vi "forceSubpanelAbort.vi"(8 "error in":errorcluster, 11 "SubPanel in":refnum<class "xceSubPanel.lvclass">) -> (0 "error out":errorcluster, 3 "SubPanel out":refnum<class "xceSubPanel.lvclass">)   [LabVIEW 2013, in "xceSubPanel.lvclass"]
doc: "Used to force if a subpanel to close its current subVI. This was added in case an unhandled error occured, and the user did not want to force a UI VI to close separately."
uses:
  xceSubPanel.lvclass
  xceSubPanel.lvclass/xceSubPanel.ctl
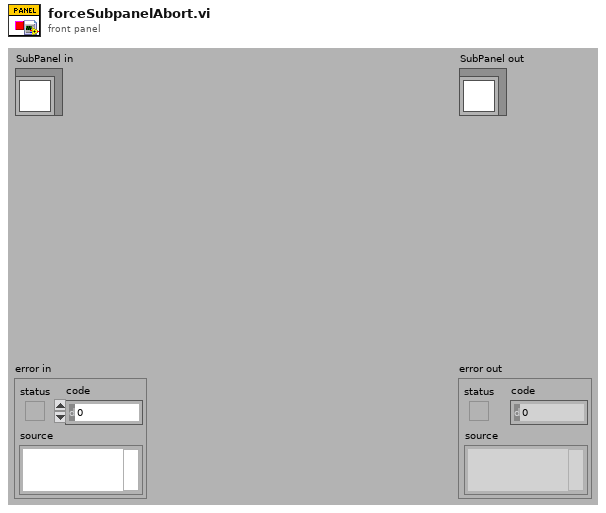
[diagram p1: front panel]
types:
  T1 = enum32{"Bad", "Idle", "Run top level", "Running"}
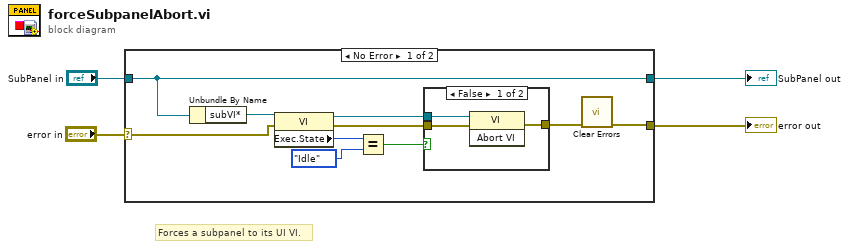
[diagram p0: block diagram]
diagram:
  # "Forces a subpanel to its UI VI."
  n1 = case shown="No Error" "error in" {
    selector: "error in" -> [w12 w20]
    tunnel: [w5 w20] -> w3
    tunnel: [w14 w19] -> w1
    tunnel: "SubPanel in" -> [w14 w19]
    frame No Error {
      n2 = Unbundle By Name(w14) -> ("subVI*"=w13:refnum<vi>)
      n3 = property class="VI"(reference=w13, error in=w12) -> (reference out=w8:refnum<vi>, error out=w7:errorcluster, "Exec.State"=w11:T1)
      n4 = Equal?(x=w11, y=T1."Idle") -> (x = y?=w9:bool)
      n5 = case shown="False" w9 {
        tunnel: w8 -> [w17 _]
        tunnel: w7 -> [w16 w18]
        tunnel: [w15 w18] -> w6
        frame False {
          n6 = invoke class="VI" method="Abort VI"(reference=w17, error in=w16) -> (error out=w15:errorcluster)  [unwired: 1 in, 2 out]
        }
        frame True {
        }
      }
      n7 = call <vilib>:"Clear Errors.vi"("error in (no error)"=w6) -> ("error out"=w5:errorcluster)  [unwired: 6 in]
    }
    frame Error {
    }
  }
  "error out" <- w3
  "SubPanel out" <- w1
